vi "Module Cleanup.vi"(8 "error in (no error)":errorcluster, 11 "HTTP Manager in":refnum<class "HTTP Manager.lvclass">) -> (0 "error out":errorcluster, 3 "HTTP Manager out":refnum<class "HTTP Manager.lvclass">)   [LabVIEW 2020, in "Volatus.lvlib" / "HTTP Manager.lvclass"]
uses:
  HTTP Manager.lvclass
  HTTP Manager.lvclass/HTTP Manager.ctl
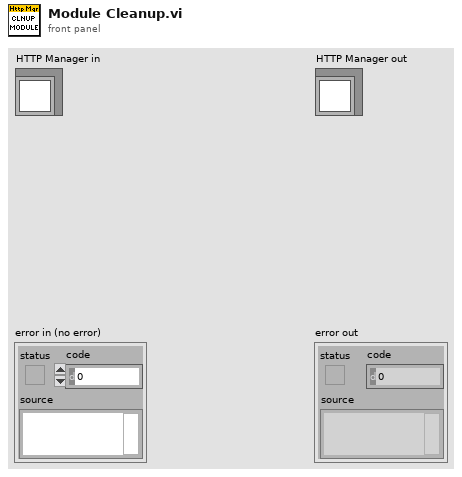
[diagram p1: front panel]
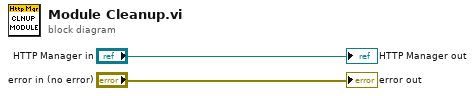
[diagram p0: block diagram]
diagram:
  "error out" <- "error in (no error)"
  "HTTP Manager out" <- "HTTP Manager in"
